vi "add_vi_by_ref.vi"(8 "error in (no error)":errorcluster, 9 "add-callers?":bool, 10 "VI Name":string, 11 "VIGraph in":refnum<class "HierarchyGraph.lvclass">) -> (0 "error out":errorcluster, 2 "vi out":refnum<class "HierarchyNode.lvclass">, 3 "VIGraph out":refnum<class "HierarchyGraph.lvclass">)   [LabVIEW 2020, in "vi-hierarchy.lvlib" / "HierarchyGraph.lvclass"]
uses:
  HierarchyGraph.lvclass
  VINode/HierarchyNode.lvclass
  HierarchyGraph.lvclass/HierarchyGraph.ctl
  <vilib>/Utility/miscctls.llb/LVMapReplaceAction.ctl
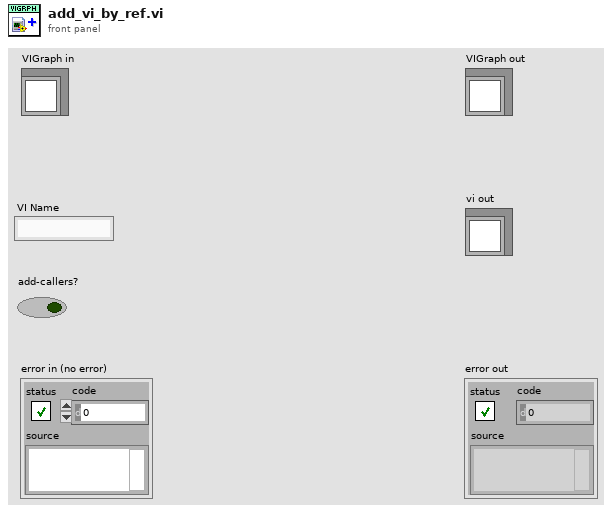
[diagram p1: front panel]
types:
  T1 = typedef "LVMapReplaceAction.ctl" = enum32{"Modify Entry only if found", "Add or Modify Entry", "Delete Entry"}
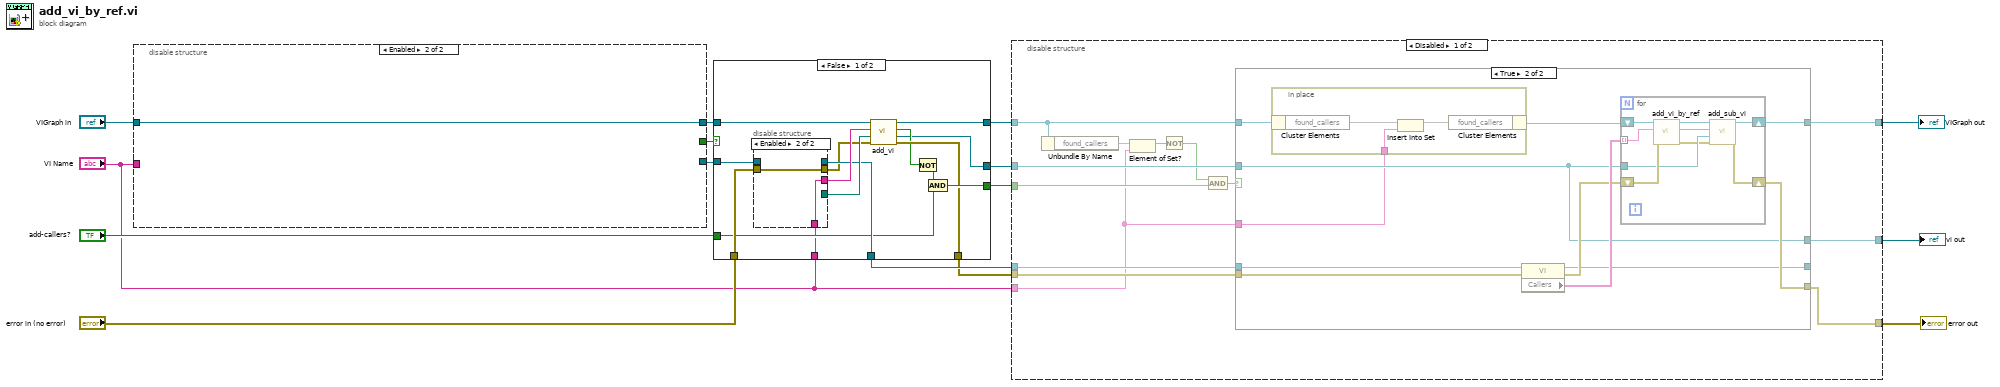
[diagram p0: block diagram]
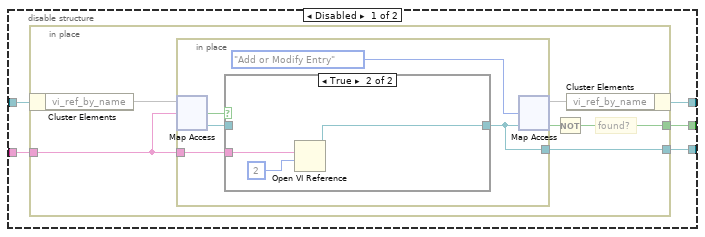
[diagram p4: hidden frame]
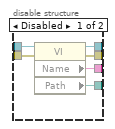
[diagram p6: hidden frame]
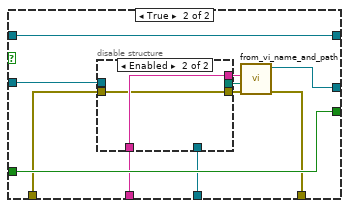
[diagram p7: hidden frame]
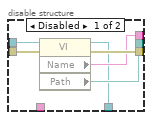
[diagram p8: hidden frame]
diagram:
  n1 = disable-structure shown="Enabled" {
    disable-tunnel: "VIGraph in" -> [w20 w36]
    disable-tunnel: [w19 w36] -> w6
    disable-tunnel: [w18 _] -> w5
    disable-tunnel: [w17 _] -> w4
    disable-tunnel: "VI Name" -> [w16 _]
    frame Disabled {
      n2 = in-place {
        in-place-border: w16 -> [w25]
        in-place-border: [w23] -> w18
        in-place-border: [w21] -> w17
        # "found?"
        n3 = in-place-cluster #1(w20) -> ("vi_ref_by_name"=w26:map{string, refnum<vi>})
        n4 = in-place {
          in-place-border: w25 -> [w30]
          in-place-border: [w27] -> w23
          n5 = in-place-map #2(w26, w25) -> (w29:refnum<vi>, w31:bool)  [unwired: 1 in]
          n6 = case shown="True" w31 {
            tunnel: w30 -> [_ w34]
            tunnel: [w32 w33] -> w27
            tunnel: w29 -> [w32 _]
            frame False {
            }
            frame True {
              n7 = Open VI Reference(vi path=w34, options=2) -> (vi reference=w33:refnum<vi>)  [unwired: 4 in, 1 out]
            }
          }
          n8 = in-place-map #2(w27, LVMapReplaceAction."Add or Modify Entry" ("action")) -> (w24:map{string, refnum<vi>}, w22:bool)  [unwired: 1 out]
        }
        n9 = Not(x=w22) -> (.not. x?=w21:bool)
        n10 = in-place-cluster #1("vi_ref_by_name"=w24) -> (w19:refnum<class "HierarchyGraph.lvclass">)
      }
    }
    frame Enabled {
    }
  }
  n11 = case shown="False" w4 {
    tunnel: "error in (no error)" -> [w49 w62]
    tunnel: [w48 w70] -> w2
    tunnel: "add-callers?" -> [w41 w69]
    tunnel: [w47 w69] -> w10
    tunnel: [w46 w64] -> w9
    tunnel: [w44 w61] -> w8
    tunnel: w6 -> [w43 w70]
    tunnel: w5 -> [w42 w65]
    tunnel: [w38 w63] -> w3
    tunnel: "VI Name" -> [w37 w60]
    frame False {
      n12 = disable-structure shown="Enabled" {
        disable-tunnel: [w57 w59] -> w51
        disable-tunnel: [w56 _] -> w50
        disable-tunnel: w49 -> [w55 w58]
        disable-tunnel: [w54 _] -> w46
        disable-tunnel: [w53 w58] -> w45
        disable-tunnel: w42 -> [w52 _]
        disable-tunnel: w37 -> [_ w59]
        frame Disabled {
          n13 = property class="VI"(reference=w52, error in=w55) -> (reference out=w54:refnum<vi>, error out=w53:errorcluster, "Name"=w57:string, "Path"=w56:path)
        }
        frame Enabled {
        }
      }
      n14 = call "add_vi.vi"("error in (no error)"=w45, "Path"=w50, "vi_name"=w51, "VIGraph in"=w43) -> ("error out"=w44:errorcluster, "VINode out"=w38:refnum<class "HierarchyNode.lvclass">, "node already included?"=w39:bool, "VIGraph out"=w48:refnum<class "HierarchyGraph.lvclass">)  [unwired: 4 in]
      n15 = Not(x=w39) -> (.not. x?=w40:bool)
      n16 = And(x=w40, y=w41) -> (x .and. y?=w47:bool)
    }
    frame True {
      n17 = disable-structure shown="Enabled" {
        disable-tunnel: [w76 w77] -> w68
        disable-tunnel: [w75 _] -> w67
        disable-tunnel: [w74 w78] -> w66
        disable-tunnel: w65 -> [w73 _]
        disable-tunnel: [w72 _] -> w64
        disable-tunnel: w62 -> [w71 w77]
        disable-tunnel: w60 -> [_ w78]
        frame Disabled {
          n18 = property class="VI"(reference=w73, error in=w71) -> (reference out=w72:refnum<vi>, error out=w76:errorcluster, "Name"=w74:string, "Path"=w75:path)
        }
        frame Enabled {
        }
      }
      n19 = call "from_vi_name_and_path.vi"("error in (no error)"=w68, "Path"=w67, "vi_name"=w66) -> ("error out"=w61:errorcluster, "VINode out"=w63:refnum<class "HierarchyNode.lvclass">)  [unwired: 7 in]
    }
  }
  n20 = disable-structure shown="Disabled" {
    disable-tunnel: [w91 w121] -> w14
    disable-tunnel: [w90 w119] -> w13
    disable-tunnel: [w89 w120] -> w12
    disable-tunnel: w10 -> [w88 _]
    disable-tunnel: w9 -> [w87 _]
    disable-tunnel: w8 -> [w86 w119]
    disable-tunnel: w3 -> [w85 w120]
    disable-tunnel: w2 -> [w84 w121]
    disable-tunnel: "VI Name" -> [w79 _]
    frame Disabled {
      n21 = Unbundle By Name(w84) -> ("found_callers"=w83:set{string})
      n22 = Element of Set?(10:w79, 11:w83) -> (3:w81:bool)
      n23 = Not(x=w81) -> (.not. x?=w80:bool)
      n24 = And(x=w80, y=w88) -> (x .and. y?=w82:bool)
      n25 = case shown="True" w82 {
        tunnel: w87 -> [w94 w102]
        tunnel: [w94 w99] -> _
        tunnel: w84 -> [w95 w98]
        tunnel: [w95 w106] -> w91
        tunnel: [w93 w103] -> w90
        tunnel: w86 -> [w93 w101]
        tunnel: [w92 w100] -> w89
        tunnel: w85 -> [w92 w100]
        tunnel: w79 -> [_ w97]
        frame False {
        }
        frame True {
          n26 = in-place {
            in-place-border: w97 -> [w107]
            n27 = in-place-cluster #3(w98) -> ("found_callers"=w109:set{string})
            n28 = Insert Into Set(10:w107, 11:w109) -> (3:w108:set{string})  [unwired: 1 out]
            n29 = in-place-cluster #3("found_callers"=w108) -> (w96:refnum<class "HierarchyGraph.lvclass">)
          }
          n30 = property class="VI"(reference=w102, error in=w101) -> (reference out=w99:refnum<vi>, error out=w104:errorcluster, "Callers"=w105:string[])
          n31 = for {
            tunnel: w105 -> [w117] mode=indexing
            shift-right: [w114] -> w106
            shift-left: w96 -> [w118]
            shift-right: [w110] -> w103
            shift-left: w104 -> [w116]
            tunnel: w100 -> [w112]
            n32 = call "add_vi_by_ref.vi"("error in (no error)"=w116, "VI Name"=w117, "VIGraph in"=w118) -> ("error out"=w111:errorcluster, "vi out"=w113:refnum<class "HierarchyNode.lvclass">, "VIGraph out"=w115:refnum<class "HierarchyGraph.lvclass">)  [unwired: 6 in]
            n33 = call "add_sub_vi.vi"("error in (no error)"=w111, "SubVI"=w112, "VI"=w113, "VIHierarchyGraph in"=w115) -> ("error out"=w110:errorcluster, "VIHierarchyGraph out"=w114:refnum<class "HierarchyGraph.lvclass">)  [unwired: 6 in]
          }
        }
      }
    }
    frame Enabled {
    }
  }
  "error out" <- w13
  "VIGraph out" <- w14
  "vi out" <- w12
